vi "Generate Send Data Command.vi"(0 "Sensor Address In":string="a", 1 "CRC (False)":bool, 5 "Measurement Type In (Normal)":i32(ring) items=["Normal", "Concurrent", "Continuous"], 7 "Send Iteration (0)":i32, 11 "Error In (No Error)":errorcluster) -> (4 "Send Command":string, 15 "Error Out":errorcluster)   [LabVIEW 2016, in "SDI-12.lvlib"]
doc: "Constructs the Send Data Command that is to be sent to a sensor in order to collect data.\n\nFor Normal and Concurrent Measurements (Regardless if Additional or CRC are enabled):\naD0!\n...\naD9!\n\nFor Continuous Measurements without CRC:\naR0!\n...\naR9!\n\nFor Continuous Measurements with CRC:\naRC0!\n...\naRC9!\n\nWhere:\na = Any valid SDI-12 address.\n0-9 = The Send Iteration.\n\nVisit http://www.sdi-12.org/ for more details on the syntax of send commands."
uses:
  SDI-12.lvlib
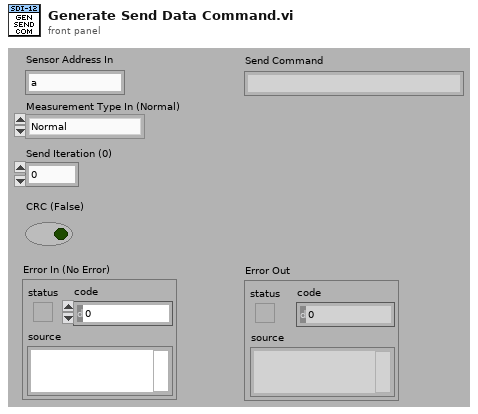
[diagram p1: front panel]
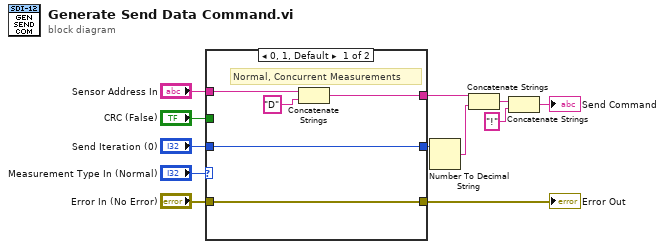
[diagram p0: block diagram]
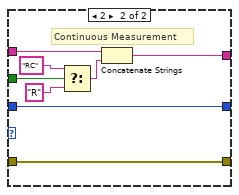
[diagram p2: hidden frame]
diagram:
  n1 = case shown="0, 1, Default" "Measurement Type In (Normal)" {
    tunnel: "Sensor Address In" -> [w17 w25]
    tunnel: "CRC (False)" -> [_ w20]
    tunnel: [w16 w24] -> w5
    tunnel: "Error In (No Error)" -> [w14 w23]
    tunnel: [w14 w23] -> w3
    tunnel: "Send Iteration (0)" -> [w13 w18]
    tunnel: [w13 w18] -> w1
    frame 0, 1, Default {
      # "Normal, Concurrent Measurements"
      n2 = Concatenate Strings(w17, "D" ("string")) -> (w16:string)
    }
    frame 2 {
      # "Continuous Measurement"
      n3 = Select(t="RC" ("string"), s=w20, f="R" ("string")) -> (s? t:f=w19:string)
      n4 = Concatenate Strings(w25, w19) -> (w24:string)
    }
  }
  "Error Out" <- w3
  n5 = Number To Decimal String(number=w1) -> (decimal integer string=w7:string)  [unwired: 1 in]
  n6 = Concatenate Strings(w5, w7) -> (w6:string)
  n7 = Concatenate Strings(w6, "!" ("string")) -> (→"Send Command":string)
